vi "State Change Core.vi"(8 "error in":errorcluster, 10 "Transition State":refnum<class "State Change Core.lvclass">, 11 "State Change Core in":refnum<class "State Change Core.lvclass">) -> (0 "error out":errorcluster, 3 "State Change Core out":refnum<class "State Change Core.lvclass">)   [LabVIEW 2021, in "State Change Core.lvlib" / "State Change Core.lvclass"]
uses:
  State Change Core.lvclass
  C:/PPLs/Design-Patterns/State Pattern/State Pattern/State Pattern/State Pattern.lvclass
  State Pattern/State Pattern.lvclass
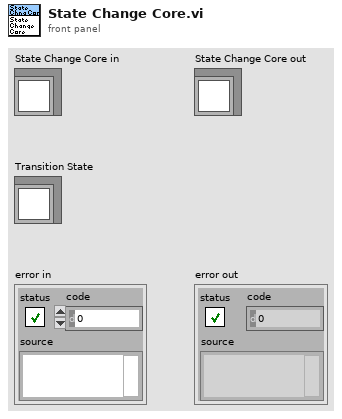
[diagram p1: front panel]
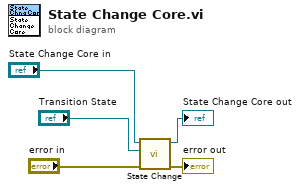
[diagram p0: block diagram]
diagram:
  n1 = call "State Change.vi"("error in"="error in", "Transition State"="Transition State", "Context in"="State Change Core in") -> ("error out"=→"error out":errorcluster, "Context out"=→"State Change Core out":refnum<class "State Change Core.lvclass">)  [unwired: 7 in]
